vi "Mutate_v1_to_v2.vi"(11 "SerializableData_v1":T2) -> (0 "error out":errorcluster, 3 "SerializableData":T1)   [LabVIEW 2019, in "Chevy Chase.lvclass"]
uses:
  Chevy Chase.lvclass
  SerializableData_v1.ctl
  SerializableData.ctl
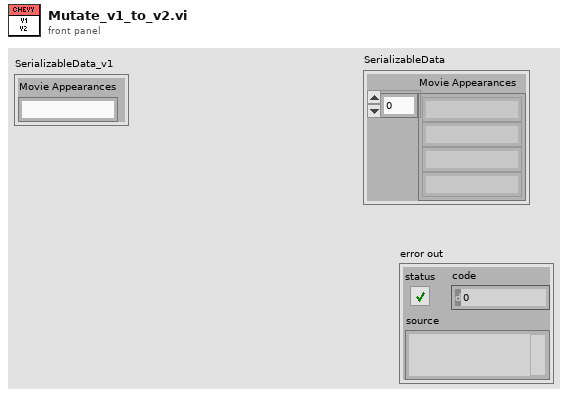
[diagram p1: front panel]
types:
  T1 = typedef "Chevy Chase.lvclass/SerializableData.ctl" = cluster{"Movie Appearances":string[]}
  T2 = typedef "Chevy Chase.lvclass/SerializableData_v1.ctl" = cluster{"Movie Appearances":string}
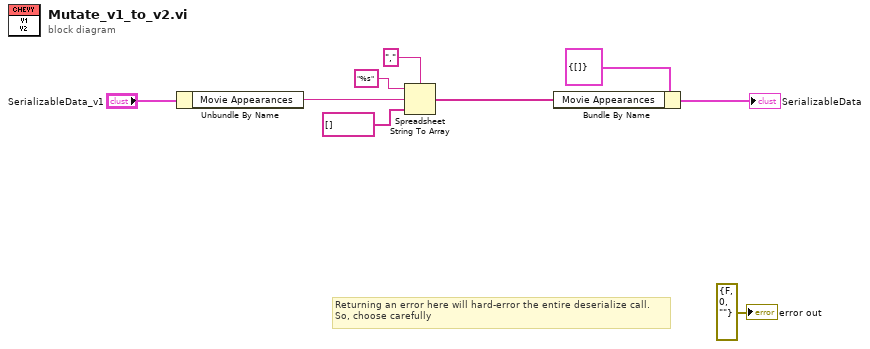
[diagram p0: block diagram]
diagram:
  # "Returning an error here will hard-error the entire deserialize call.\nSo, choose carefully"
  n1 = Unbundle By Name("SerializableData_v1") -> ("Movie Appearances"=w6:string)
  n2 = Spreadsheet String To Array(delimiter (Tab)=",", format string="%s", spreadsheet string=w6, array type (2D Dbl)=string[] []) -> (array=w2:string[])
  n3 = Bundle By Name(cluster=T1 {"Movie Appearances"=[]} ("SerializableData"), "Movie Appearances"=w2) -> (→"SerializableData":T1)
  "error out" <- errorcluster {"status"=FALSE, "code"=0, "source"=""} ("error out")
